vi "LLDP.vi"(10 "Data in":string="\u0001Â\u0000\u0000\u000e\u0000\u001b\u001b+÷\u001bÌ\u0002\u0006\u0007pn-io\u0004\t\u0007port-001\u0006\u0002\u0000\u0014\u0010\u0014\u0005\u0001À¨dU\u0002\u0000\u0000\u0000\u0002\b+\u0006\u0001\u0004\u0001Ànþ\u0018\u0000\u000eÏ\u0001\u0000\u0000\u0000é\u0000\u0000\u0000\u0000\u0000\u0000\u0000x\u0000\u0000\u0000\u0000\u0000\u0000\u0000\u0000þ\b\u0000\u000eÏ\u0002\u0000\u0000\u0000\u0000þ\n\u0000\u000eÏ\u0005\u0000\u001b\u001b+÷\u001aþ\t\u0000\u0012\u000f\u0001\u0003l\u0000\u0000\u0010\u0000\u0000") -> (2 "LLDP packet":bool, 3 "LLDP":T1)   [LabVIEW 2017]
uses:
  TypeDefs/control_packet_header_ethernet.ctl
  TypeDefs/LLDP.ctl
panel:
  out "Time to live":i16
  out "ethernet header":T2 {"destination MAC address"."?" format="%02x"; "destination MAC address"."?" format="%02x"; "destination MAC address"."?" format="%02x"; "destination MAC address"."?" format="%02x"; "destination MAC address"."?" format="%02x"; "destination MAC address"."?" format="%02x"; "source MAC address"."?" format="%02x"; "source MAC address"."?" format="%02x"; "source MAC address"."?" format="%02x"; "source MAC address"."?" format="%02x"; "source MAC address"."?" format="%02x"; "source MAC address"."?" format="%02x"; "length / type" format="%04x"}
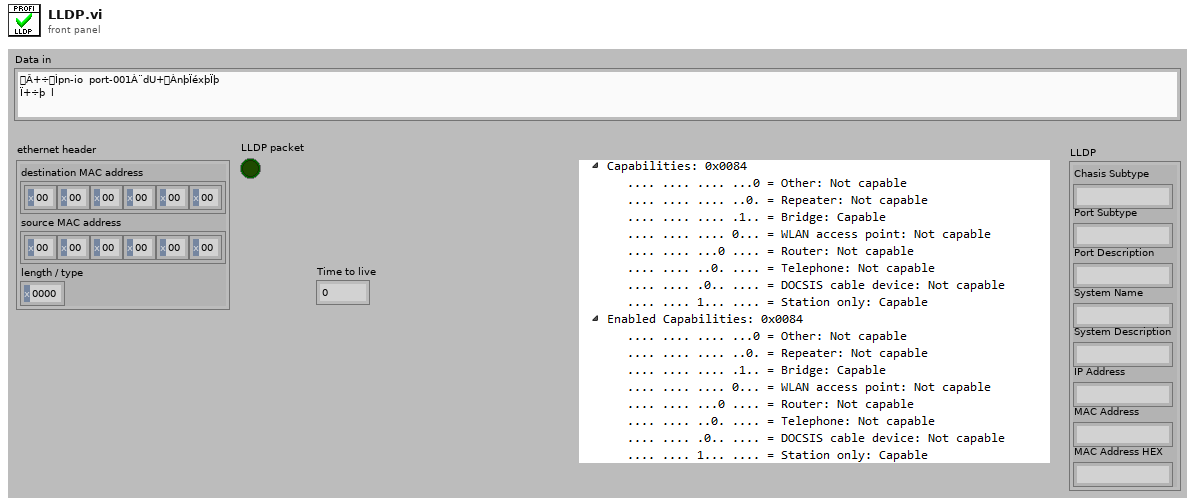
[diagram p1: front panel]
types:
  T1 = typedef "LLDP.ctl" = cluster{"Chasis Subtype":string, "Port Subtype":string, "Port Description":string, "System Name":string, "System Description":string, "IP Address":string, "MAC Address":string, "MAC Address HEX":string}
  T2 = typedef "control_packet_header_ethernet.ctl" = cluster{"destination MAC address":cluster{u8, u8, u8, u8, u8, u8}, "source MAC address":cluster{u8, u8, u8, u8, u8, u8}, "length / type":u16}
  T3 = enum16{"Check Header", "Chasis Subtype", "Port Subtype", "Time to live", "Port Description", "System Name", "System Description", "Capabilities", "Managment Address"}
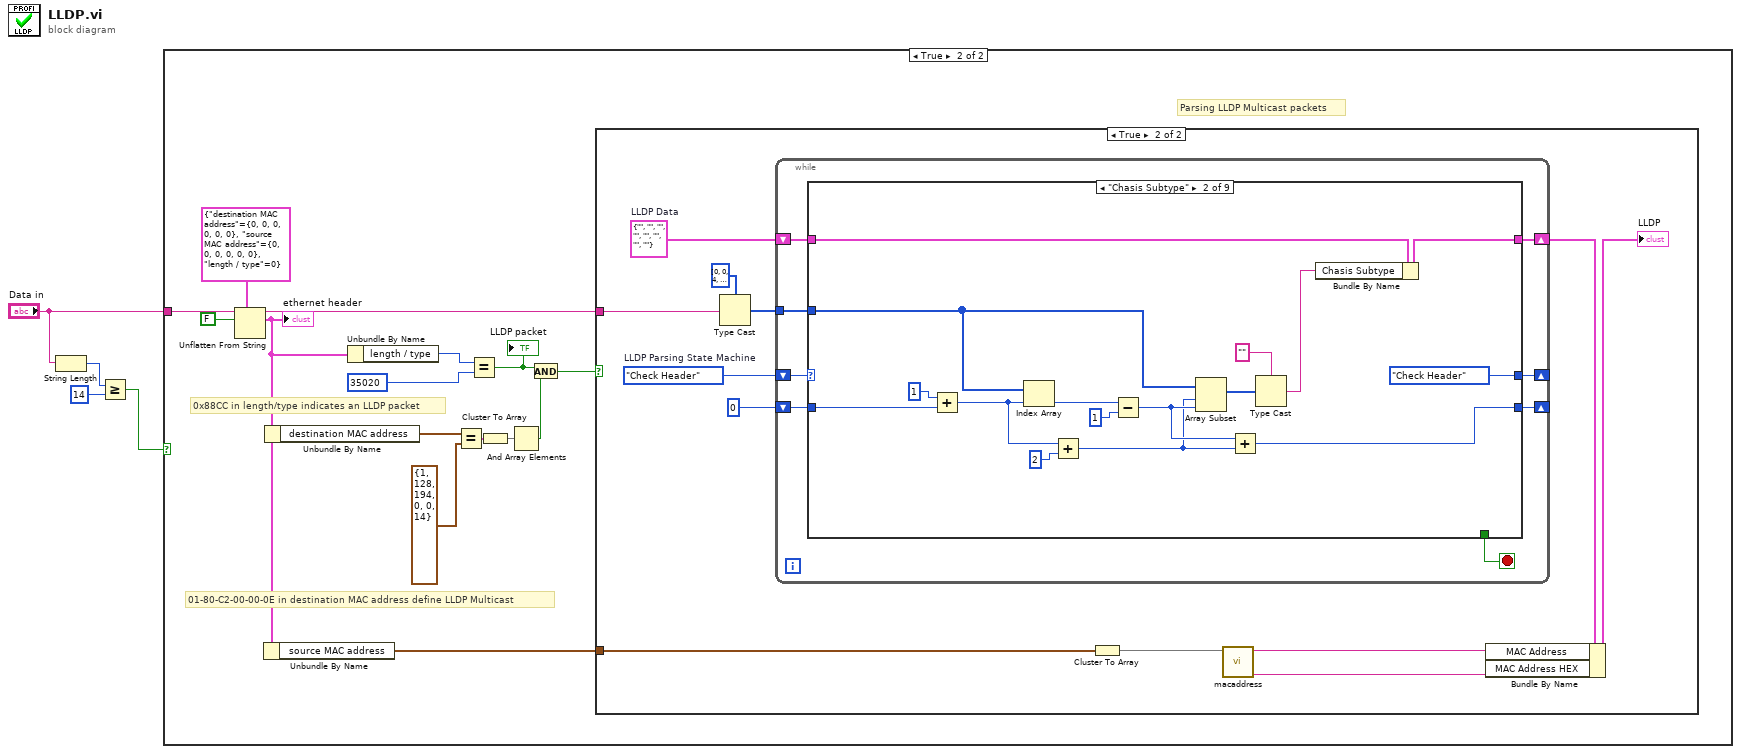
[diagram p0: block diagram]
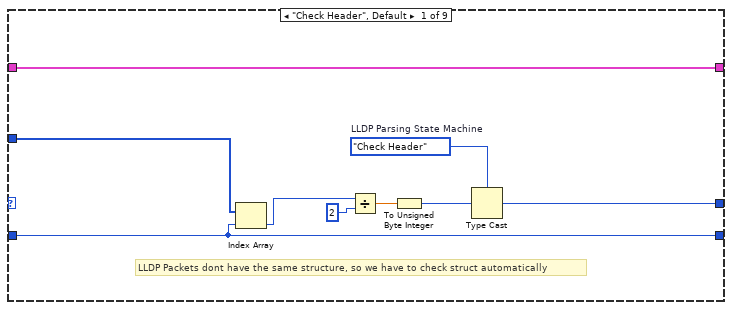
[diagram p4: hidden frame]
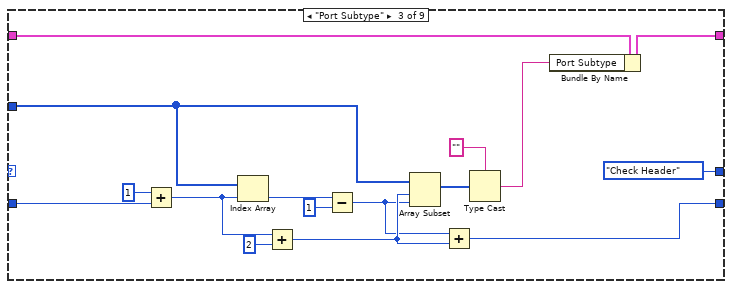
[diagram p5: hidden frame]
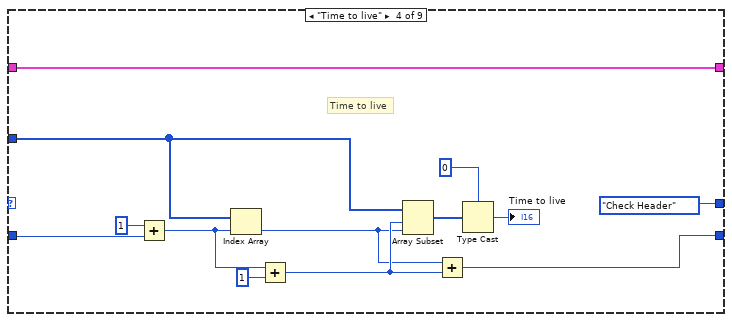
[diagram p6: hidden frame]
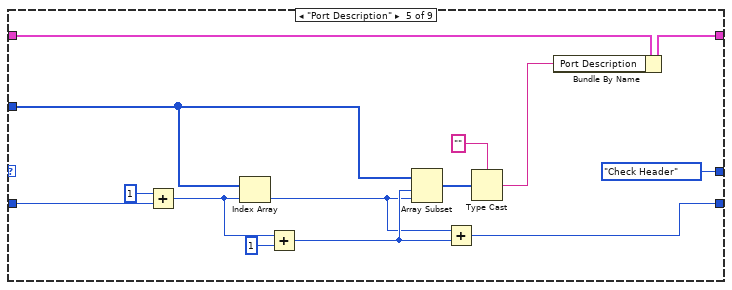
[diagram p7: hidden frame]
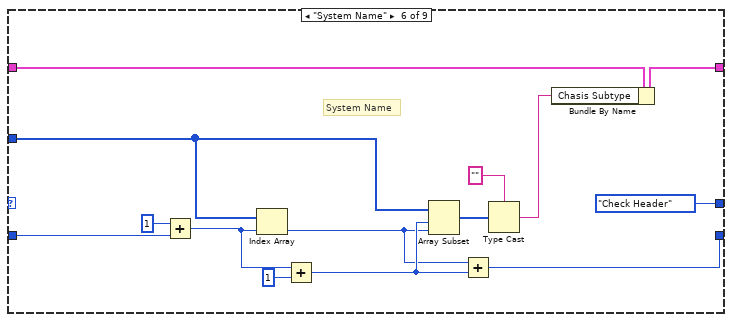
[diagram p8: hidden frame]
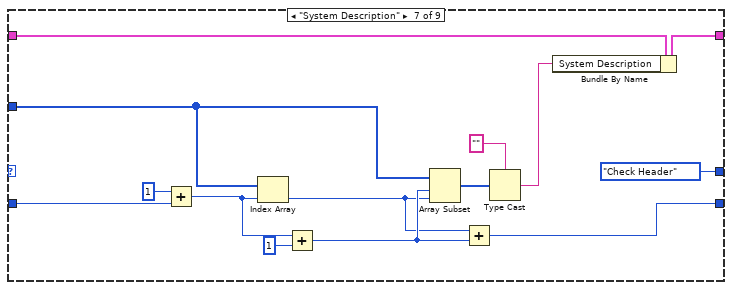
[diagram p9: hidden frame]
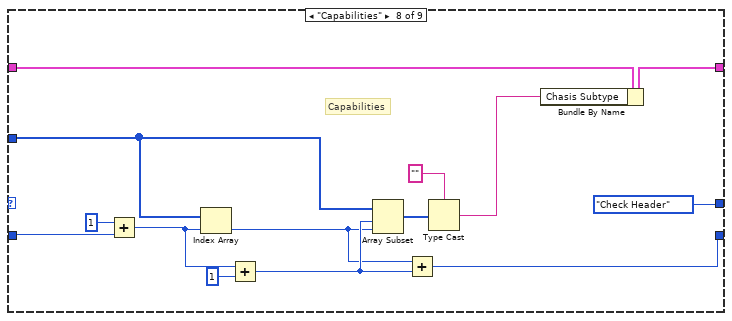
[diagram p10: hidden frame]
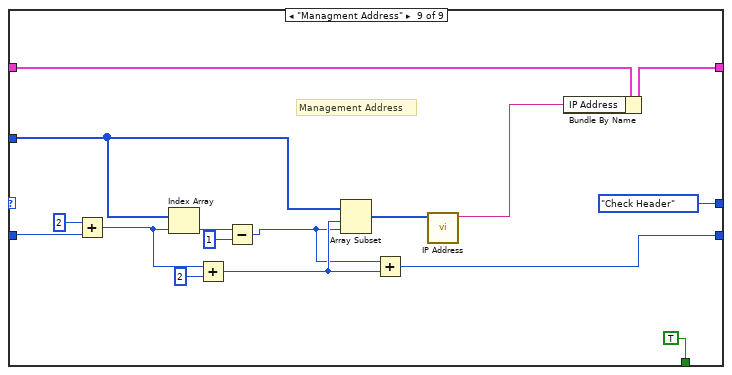
[diagram p11: hidden frame]
diagram:
  n1 = String Length(string="Data in") -> (length=w3:i32)
  n2 = Greater Or Equal?(x=w3, y=14) -> (x >= y?=w2:bool)
  n3 = case shown="True" w2 {
    tunnel: "Data in" -> [_ w14]
    frame False {
    }
    frame True {
      # "Parsing LLDP Multicast packets"
      # "01-80-C2-00-00-0E in destination MAC address define LLDP Multicast"
      # "0x88CC in length/type indicates an LLDP packet"
      n4 = Unflatten From String(type=T2 {"destination MAC address"={0, 0, 0, 0, 0, 0}, "source MAC address"={0, 0, 0, 0, 0, 0}, "length / type"=0} ("ethernet header"), binary string=w14, data includes array or string size? (T)=FALSE) -> (rest of the binary string=w15:string, value=w6:T2)  [unwired: 2 in, 1 out]
      "ethernet header" <- w6
      n5 = Unbundle By Name(w6) -> ("source MAC address"=w5:cluster{u8, u8, u8, u8, u8, u8})
      n6 = Unbundle By Name(w6) -> ("destination MAC address"=w7:cluster{u8, u8, u8, u8, u8, u8})
      n7 = Unbundle By Name(w6) -> ("length / type"=w17:u16)
      n8 = Equal?(x=w7, y=cluster{u8, u8, u8, u8, u8, u8} {1, 128, 194, 0, 0, 14}) -> (x = y?=w12:cluster{bool, bool, bool, bool, bool, bool})
      n9 = Equal?(x=w17, y=u16 35020) -> (x = y?=w9:bool)
      "LLDP packet" <- w9
      n10 = Cluster To Array(cluster=w12) -> (array=w11:bool[])
      n11 = And Array Elements(Boolean array=w11) -> (logical AND=w8:bool)
      n12 = And(x=w9, y=w8) -> (x .and. y?=w10:bool)
      n13 = case shown="True" w10 {
        tunnel: w15 -> [_ w31]
        tunnel: w5 -> [_ w30]
        frame False {
        }
        frame True {
          w23 = T3."Check Header"  # LLDP Parsing State Machine
          w24 = T1 {"Chasis Subtype"="", "Port Subtype"="", "Port Description"="", "System Name"="", "System Description"="", "IP Address"="", "MAC Address"="", "MAC Address HEX"=""}  # LLDP Data
          n14 = Type Cast(type=u8[] [0, 0, 4, 0, 1, 0, 1, 0, 0, 0, 0, 0, 0, 0, 0, 0, 0, 0, 0, 0, 0, 0, 0, 0, 1, 0, 0, 0] ("Byte Array"), x=w31) -> (*(type *) &x=w28:u8[])
          n15 = while {
            tunnel: w28 -> [w39]
            shift-right: [w36] -> _
            shift-left: w23 -> [w38]
            shift-right: [w35] -> _
            shift-left: 0 ("index") -> [w37]
            shift-right: [w32] -> w22
            shift-left: w24 -> [w33]
            stop <- w34 stop-if-true
            n16 = case shown="\"Chasis Subtype\"" w38 {
              tunnel: w39 -> [w48 w57 w71 w87 w101 w114 w128 w144 w161]
              tunnel: w37 -> [w47 w63 w70 w86 w100 w113 w127 w143 w160]
              tunnel: [w40 T3."Check Header" ("LLDP Parsing State Machine") T3."Check Header" ("LLDP Parsing State Machine") T3."Check Header" ("LLDP Parsing State Machine") T3."Check Header" ("LLDP Parsing State Machine") T3."Check Header" ("LLDP Parsing State Machine") T3."Check Header" ("LLDP Parsing State Machine") T3."Check Header" ("LLDP Parsing State Machine") T3."Check Header" ("LLDP Parsing State Machine")] -> w36
              tunnel: [w47 w53 w69 w85 w99 w112 w126 w142 w159] -> w35
              tunnel: [_ _ _ _ _ _ _ _ TRUE] -> w34
              tunnel: w33 -> [w43 w52 w67 w81 w96 w110 w124 w138 w152]
              tunnel: [w43 w50 w66 w81 w95 w109 w123 w137 w151] -> w32
              frame "Check Header", Default {
                w41 = T3."Check Header"  # LLDP Parsing State Machine
                # "LLDP Packets dont have the same structure, so we have to check struct automatically"
                n17 = Index Array(array=w48, index=w47) -> (element=w46:u8)
                n18 = Divide(x=w46, y=u8 2) -> (x/y=w44:dbl)
                n19 = To Unsigned Byte Integer(number=w44) -> (unsigned 8bit integer=w42:u8)
                n20 = Type Cast(type=w41, x=w42) -> (*(type *) &x=w40:T3)
              }
              frame "Chasis Subtype" {
                n21 = Add(x=1, y=w63) -> (x+y=w59:i32)
                n22 = Index Array(array=w57, index=w59) -> (element=w61:u8)
                n23 = Add(x=w59, y=2) -> (x+y=w54:i32)
                n24 = Subtract(x=w61, y=u8 1) -> (x-y=w55:u8)
                n25 = Array Subset(array=w57, index=w54, length=w55) -> (w56:u8[])
                n26 = Add(x=w55, y=w54) -> (x+y=w53:i32)
                n27 = Type Cast(type="", x=w56) -> (*(type *) &x=w51:string)
                n28 = Bundle By Name(cluster=w52, "Chasis Subtype"=w51) -> (w50:T1)
              }
              frame "Port Subtype" {
                n29 = Add(x=1, y=w70) -> (x+y=w76:i32)
                n30 = Index Array(array=w71, index=w76) -> (element=w74:u8)
                n31 = Add(x=w76, y=2) -> (x+y=w80:i32)
                n32 = Subtract(x=w74, y=u8 1) -> (x-y=w79:u8)
                n33 = Array Subset(array=w71, index=w80, length=w79) -> (w78:u8[])
                n34 = Add(x=w79, y=w80) -> (x+y=w69:i32)
                n35 = Type Cast(type="", x=w78) -> (*(type *) &x=w65:string)
                n36 = Bundle By Name(cluster=w67, "Port Subtype"=w65) -> (w66:T1)
              }
              frame "Time to live" {
                # "Time to live"
                n37 = Add(x=1, y=w86) -> (x+y=w90:i32)
                n38 = Index Array(array=w87, index=w90) -> (element=w88:u8)
                n39 = Add(x=w90, y=1) -> (x+y=w93:i32)
                n40 = Array Subset(array=w87, index=w93, length=w88) -> (w92:u8[])
                n41 = Add(x=w88, y=w93) -> (x+y=w85:i32)
                n42 = Type Cast(type=i16 0, x=w92) -> (*(type *) &x=→"Time to live":i16)
              }
              frame "Port Description" {
                n43 = Add(x=1, y=w100) -> (x+y=w104:i32)
                n44 = Index Array(array=w101, index=w104) -> (element=w102:u8)
                n45 = Add(x=w104, y=1) -> (x+y=w107:i32)
                n46 = Array Subset(array=w101, index=w107, length=w102) -> (w106:u8[])
                n47 = Add(x=w102, y=w107) -> (x+y=w99:i32)
                n48 = Type Cast(type="", x=w106) -> (*(type *) &x=w94:string)
                n49 = Bundle By Name(cluster=w96, "Port Description"=w94) -> (w95:T1)
              }
              frame "System Name" {
                # "System Name"
                n50 = Add(x=1, y=w113) -> (x+y=w118:i32)
                n51 = Index Array(array=w114, index=w118) -> (element=w116:u8)
                n52 = Add(x=w118, y=1) -> (x+y=w121:i32)
                n53 = Array Subset(array=w114, index=w121, length=w116) -> (w120:u8[])
                n54 = Add(x=w116, y=w121) -> (x+y=w112:i32)
                n55 = Type Cast(type="", x=w120) -> (*(type *) &x=w108:string)
                n56 = Bundle By Name(cluster=w110, "Chasis Subtype"=w108) -> (w109:T1)
              }
              frame "System Description" {
                n57 = Add(x=1, y=w127) -> (x+y=w132:i32)
                n58 = Index Array(array=w128, index=w132) -> (element=w130:u8)
                n59 = Add(x=w132, y=1) -> (x+y=w135:i32)
                n60 = Array Subset(array=w128, index=w135, length=w130) -> (w134:u8[])
                n61 = Add(x=w130, y=w135) -> (x+y=w126:i32)
                n62 = Type Cast(type="", x=w134) -> (*(type *) &x=w122:string)
                n63 = Bundle By Name(cluster=w124, "System Description"=w122) -> (w123:T1)
              }
              frame "Capabilities" {
                # "Capabilities"
                n64 = Add(x=1, y=w143) -> (x+y=w147:i32)
                n65 = Index Array(array=w144, index=w147) -> (element=w145:u8)
                n66 = Add(x=w147, y=1) -> (x+y=w149:i32)
                n67 = Array Subset(array=w144, index=w149, length=w145) -> (w141:u8[])
                n68 = Add(x=w145, y=w149) -> (x+y=w142:i32)
                n69 = Type Cast(type="", x=w141) -> (*(type *) &x=w136:string)
                n70 = Bundle By Name(cluster=w138, "Chasis Subtype"=w136) -> (w137:T1)
              }
              frame "Managment Address" {
                # "Management Address"
                n71 = Add(x=2, y=w160) -> (x+y=w163:i32)
                n72 = Index Array(array=w161, index=w163) -> (element=w158:u8)
                n73 = Add(x=w163, y=2) -> (x+y=w165:i32)
                n74 = Subtract(x=w158, y=u8 1) -> (x-y=w156:u8)
                n75 = Array Subset(array=w161, index=w165, length=w156) -> (w154:u8[])
                n76 = Add(x=w156, y=w165) -> (x+y=w159:i32)
                n77 = call "IP Address.vi"("Data"=w154) -> ("IP Address"=w150:string)  [unwired: 10 in]
                n78 = Bundle By Name(cluster=w152, "IP Address"=w150) -> (w151:T1)
              }
            }
          }
          n79 = Cluster To Array(cluster=w30) -> (array=w26:u8[])
          n80 = call "macaddress.vi"("source MAC address"=w26) -> ("MAC Address HEX"=w20:string, "MAC Address"=w21:string)  [unwired: 8 in]
          n81 = Bundle By Name(cluster=w22, "MAC Address"=w21, "MAC Address HEX"=w20) -> (→"LLDP":T1)
        }
      }
    }
  }
